vi "Acquire CSV.vi"(8 "error in (no error)":errorcluster, 10 "DATA IN":refnum<queue>, 11 "Hardware Resources in":T1={"State"=enum."Idle S3DK", "Settings"="", "Online"=FALSE, "S3DK"={"Signals"={"Phasor"=[], "Analog"=[], "Digital"=[]}}, "CSV"={"Index"=0, "Parcel Length"=0, "EOF?"=FALSE, "Config"={"Mode"=enum."Full timestamp", "delimiter (\\t)"="\t", "Path"=path "", "Rectangular?"=FALSE}}}) -> (0 "error out":errorcluster, 3 "Hardware Resources out":T1={"State"=enum."Idle S3DK", "Settings"="", "Online"=FALSE, "S3DK"={"Signals"={"Phasor"=[], "Analog"=[], "Digital"=[]}}, "CSV"={"Index"=0, "Parcel Length"=0, "EOF?"=FALSE, "Config"={"Mode"=enum."Full timestamp", "delimiter (\\t)"="\t", "Path"=path "", "Rectangular?"=FALSE}}})   [LabVIEW 2017, in "Acquisition.lvlib"]
doc: "Perform the acquisition. Replace the contents of this diagram with calls to acquisition hardware."
uses:
  Acquisition.lvlib
  Acquisition Settings.ctl
  Acquisition State.ctl
  support/libs/CSV Reader/Mode CSV reader.ctl
  support/libs/PMU Buffer/Buffer DATA cluster.ctl
  support/libs/PMU Buffer/PMU data buffer.lvlib
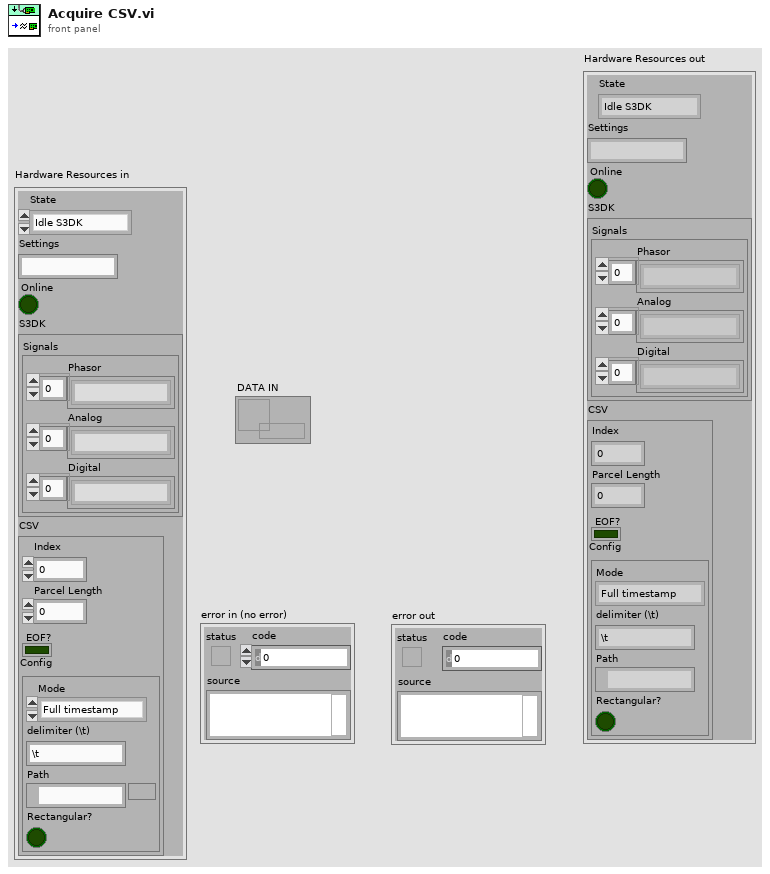
[diagram p1: front panel]
types:
  T1 = typedef "Acquisition.lvlib/Acquisition Settings.ctl" = cluster{"State":T2, "Settings":string, "Online":bool, "S3DK":cluster{"Signals":cluster{"Phasor":string[], "Analog":string[], "Digital":string[]}}, "CSV":cluster{"Index":i32, "Parcel Length":i32, "EOF?":bool, "Config":cluster{"Mode":T3, "delimiter (\\t)":string, "Path":path, "Rectangular?":bool}}}
  T2 = typedef "Acquisition.lvlib/Acquisition State.ctl" = enum16{"Idle", "Idle S3DK", "Acquiring S3DK", "Idle CSV", "Acquiring CSV"}
  T3 = typedef "Mode CSV reader.ctl" = enum16{"Full timestamp", "Relative Time", "Seconds Time", "Nanoseconds Time"}
  T4 = typedef "PMU data buffer.lvlib/Buffer DATA cluster.ctl" = cluster{timestamp, csg[], sgl[]}
  T5 = cluster{"Mode":T3, "delimiter (\\t)":string, "Path":path, "Rectangular?":bool}
  T6 = cluster{"default value 1":timestamp, "Complex":cdb[], "Analog":dbl[]}
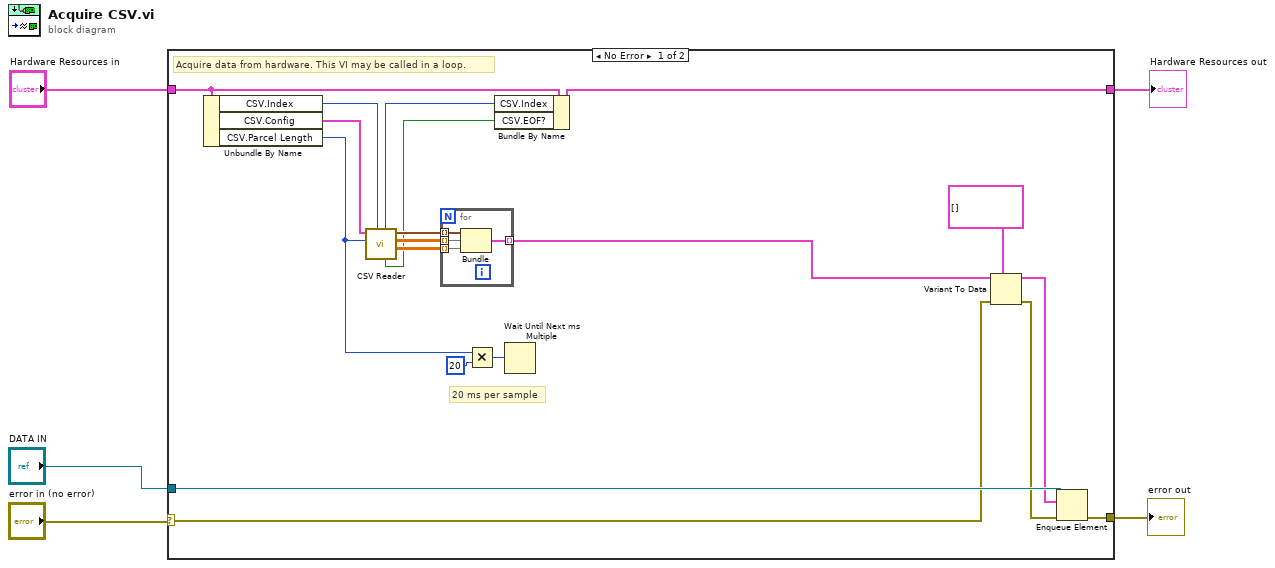
[diagram p0: block diagram]
diagram:
  n1 = case shown="No Error" "error in (no error)" {
    selector: "error in (no error)" -> [w11 w29]
    tunnel: [w23 w29] -> w4
    tunnel: "Hardware Resources in" -> [w19 w30]
    tunnel: [w18 w30] -> w2
    tunnel: "DATA IN" -> [w24 _]
    frame No Error {
      # "Acquire data from hardware. This VI may be called in a loop."
      # "20 ms per sample"
      n2 = Unbundle By Name(w19) -> ("CSV.Index"=w10:i32, "CSV.Config"=w6:T5, "CSV.Parcel Length"=w7:i32)
      n3 = call "CSV Reader.vi"("Index in"=w10, "Parcel Length"=w7, "Config"=w6) -> ("Analog"=w12:dbl[][], "Complex"=w13:cdb[][], "Timestamps"=w14:timestamp[], "EOF?"=w8:bool, "Index out"=w9:i32)  [unwired: 4 in]
      n4 = for {
        tunnel: w13 -> [w27] mode=indexing
        tunnel: w12 -> [w26] mode=indexing
        tunnel: w14 -> [w28] mode=indexing
        tunnel: [w25] -> w15 mode=indexing
        n5 = Bundle("default value 1"=w28, "Complex"=w27, "Analog"=w26) -> (w25:T6)  [unwired: 1 in]
      }
      n6 = Multiply(x=w7, y=20) -> (x*y=w16:i32)
      n7 = Bundle By Name(cluster=w19, "CSV.Index"=w9, "CSV.EOF?"=w8) -> (w18:T1)
      n8 = Wait Until Next ms Multiple(millisecond multiple=w16) -> ()  [unwired: 1 out]
      n9 = Variant To Data(error in=w11, type=T4[] [], Variant=w15) -> (data=w21:T4[], error out=w20:errorcluster)
      n10 = Enqueue Element(queue=w24, element=w21, error in (no error)=w20) -> (error out=w23:errorcluster)  [unwired: 1 in, 2 out]
    }
    frame Error {
    }
  }
  "Hardware Resources out" <- w2
  "error out" <- w4
